vi "API - Close Module.vi"(8 "Error In":errorcluster) -> (0 "Error Out":errorcluster)   [LabVIEW 2023, in "Error Manager.lvlib"]
doc: "Closes the ErrorHandler Main VI (the asynchronous module).\n\nRecommended use: Call this VI during app shutdown, after all other shutdown operations have been completed (for example, after all other asynchronous modules have been stopped). This enables the Error Manager to log any errors that may happen during app shutdown.\n\nError in behaviour: This VI executes even if 'error in' contains an error."
uses:
  Error Manager.lvlib
  MHL Queue/Command (enum).ctl
  MHL Queue/MHL Queue.lvlib
panel:
  # "Development\nControls or indicators that are useful for development or testing, but which are not outputs of the VI."
  # "Input\nInputs to the VI"
  # "Output\nOutputs of the VI"
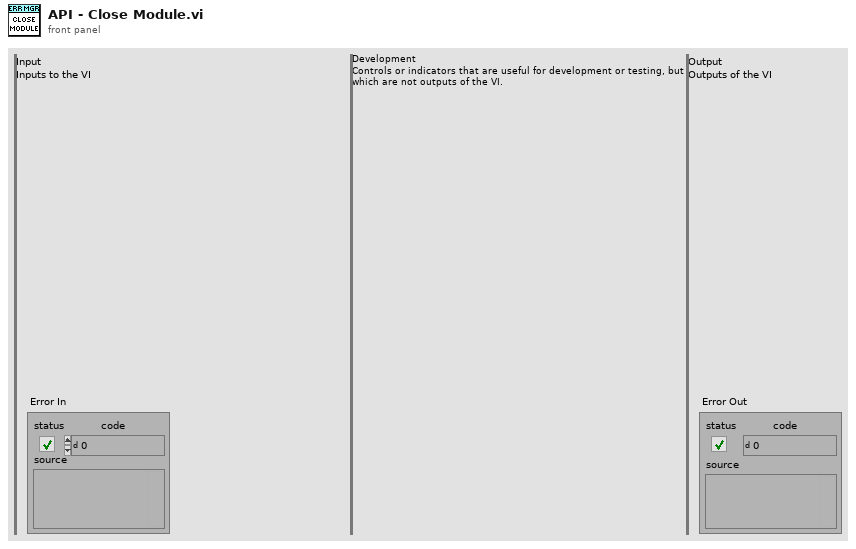
[diagram p1: front panel]
types:
  T1 = typedef "Error Manager.lvlib/MHL Queue.lvlib/Command (enum).ctl" = enum16{"Init Module", "Close Module", "Internal Error", "Create Error Log File", "Show Front Panel", "Handle Error", "Refresh MCL", "MCL Value Change", "Mark Error As Read", "Mark All Errors As Read", "Change Display Order", "One-Second Interval Expired"}
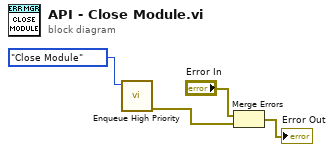
[diagram p0: block diagram]
diagram:
  n1 = call "Enqueue High Priority.vi"(11:Command_(enum)."Close Module" ("Command")) -> (0:w2:errorcluster)  [unwired: 10 in]
  n2 = Merge Errors("Error In", w2) -> (→"Error Out":errorcluster)
